vi "test_resetting_iter.vi"() -> ()   [LabVIEW 2017]
uses:
  <vilib>/rvi/Emulation/niFpgaGetClockAttributes.vi
  <vilib>/rvi/Emulation/niFpgaSctlEmulationGetInTimedLoop.vi
  <vilib>/rvi/Emulation/niFpgaEmulationReportErrorSimple.vi
  <vilib>/rvi/Emulation/niFpgaCriticalErrorInLSC.vi
  libimaging-cs.lvlib
panel:
  in  "Numeric":i32
  out "Array 2":bool[](array[boolean])
  out "Array":i16[](array[numeric])
  in  "N":i16
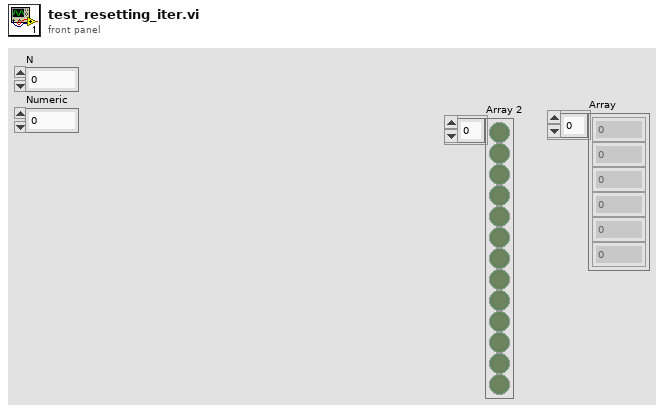
[diagram p1: front panel]
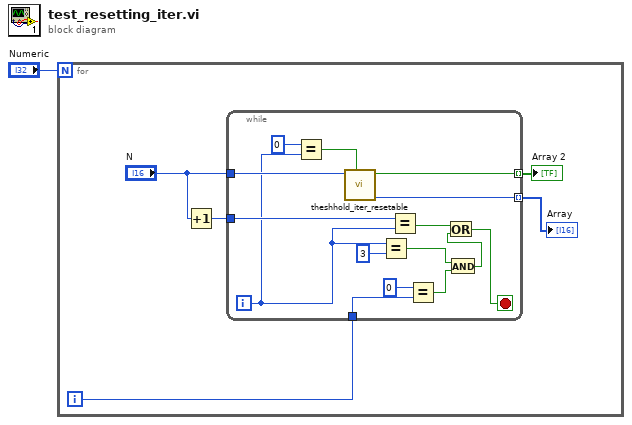
[diagram p0: block diagram]
diagram:
  n1 = for {
    N: "Numeric" -> [_]
    i -> [w3]
    n2 = Increment(x="N") -> (x+1=w2:i16)
    n3 = while {
      tunnel: [w21] -> w6 mode=indexing
      tunnel: [w20] -> w5 mode=indexing
      tunnel: "N" -> [w19]
      tunnel: w3 -> [w18]
      tunnel: w2 -> [w10]
      i -> [w9]
      stop <- w11 stop-if-true
      n4 = Equal?(x=0, y=w9) -> (x = y?=w7:bool)
      n5 = call "theshhold_iter_resetable.vi"("reset"=w7, "N"=w19) -> ("iter"=w21:i16, "Boolean"=w20:bool)  [unwired: 8 in]
      n6 = Equal?(x=w9, y=3) -> (x = y?=w14:bool)
      n7 = Equal?(x=w10, y=w9) -> (x = y?=w13:bool)
      n8 = Equal?(x=0, y=w18) -> (x = y?=w15:bool)
      n9 = And(x=w14, y=w15) -> (x .and. y?=w12:bool)
      n10 = Or(x=w13, y=w12) -> (x .or. y?=w11:bool)
    }
    "Array" <- w6
    "Array 2" <- w5
  }
